vi "Pre-Build Custom Action.vi"() -> (0 "error out":errorcluster)   [LabVIEW 2021]
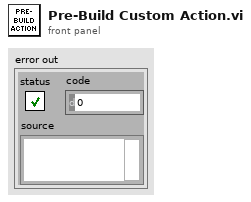
[diagram p1: front panel]
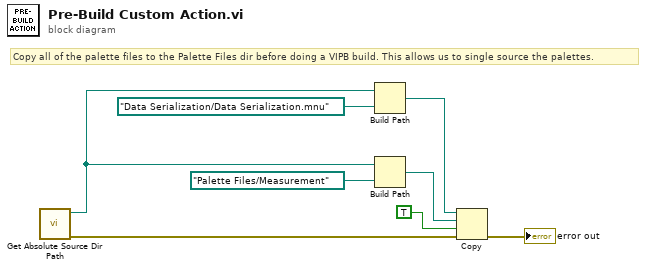
[diagram p0: block diagram]
diagram:
  # "Copy all of the palette files to the Palette Files dir before doing a VIPB build. This allows us to single source the palettes."
  n1 = call "Get Absolute Source Dir Path.vi"() -> ("error out"=w2:errorcluster, "source dir"=w3:path)  [unwired: 10 in]
  n2 = Build Path(base path=w3, name or relative path=path "Data Serialization/Data Serialization.mnu" ("source path")) -> (appended path=w6:path)
  n3 = Build Path(base path=w3, name or relative path=path "Palette Files/Measurement") -> (appended path=w7:path)
  n4 = Copy(8:w2, 9:TRUE ("overwrite (F)"), 10:w7, 11:w6) -> (0:→"error out":errorcluster)  [unwired: 1 in, 2 out]
